vi "create_full_request_data.vi"(0 "llm_ollama_embedding in":refnum<class "llm_ollama_embedding.lvclass">, 5 "data":refnum<class "abstract_message_base.lvclass">[](array[class]), 11 "error in (no error)":errorcluster) -> (4 "llm_ollama_embedding out":refnum<class "llm_ollama_embedding.lvclass">, 6 "request_data":T1[](array[typedef]), 15 "error out":errorcluster)   [LabVIEW 2020, in "llm_ollama_embedding.lvclass"]
uses:
  llm_ollama_embedding.lvclass
  abstract_message_base/abstract_message_base.lvclass
  utils/request_Data.ctl
  llm_ollama_embedding.lvclass/llm_ollama_embedding.ctl
  message_text/message_text.lvclass
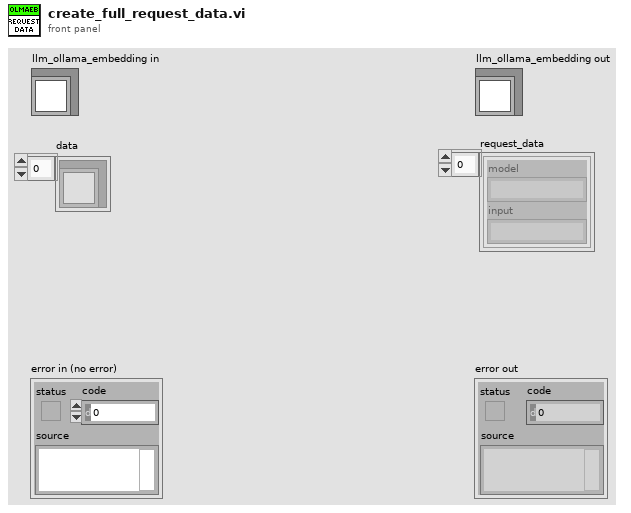
[diagram p1: front panel]
types:
  T1 = typedef "llm_ollama_embedding.lvclass/request_Data.ctl" = cluster{"model":string, "input":string}
  T2 = typedef "message_text.lvclass/message.ctl" = cluster{"role":string, "content":string[]}
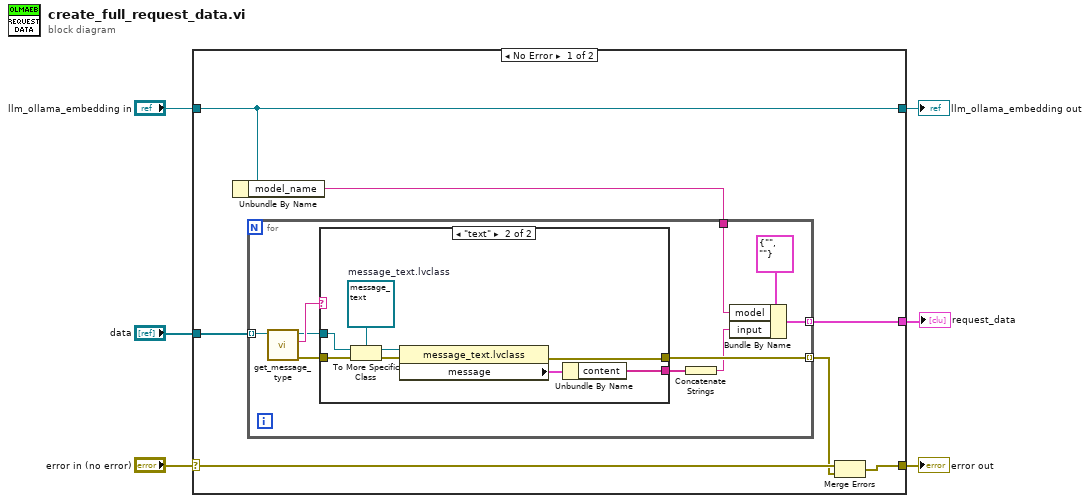
[diagram p0: block diagram]
diagram:
  n1 = case shown="No Error" "error in (no error)" {
    selector: "error in (no error)" -> [w13 w34]
    tunnel: [w10 w34] -> w5
    tunnel: [w11 w33] -> w3
    tunnel: "llm_ollama_embedding in" -> [w11 w33]
    tunnel: "data" -> [w12 _]
    tunnel: [w7 _] -> w1
    frame No Error {
      n2 = Unbundle By Name(w11) -> ("model_name"=w8:string)
      n3 = for {
        tunnel: w12 -> [w23] mode=indexing
        tunnel: [w19] -> w9 mode=indexing
        tunnel: w8 -> [w17]
        tunnel: [w14] -> w7 mode=indexing
        n4 = call-dynamic "get_message_type.vi"("abstract_message_base in"=w23) -> ("error out"=w20:errorcluster, "Type"=w22:string, "abstract_message_base out"=w21:refnum<class "abstract_message_base.lvclass">)  [unwired: 8 in]
        n5 = case shown="\"text\"" w22 {
          tunnel: w21 -> [_ w31]
          tunnel: w20 -> [w24 w32]
          tunnel: [w24 w27] -> w19
          tunnel: [_ w25] -> w18
          frame Default {
          }
          frame "text" {
            w30 = refnum<class "message_text.lvclass"> refnum  # message_text.lvclass
            n6 = To More Specific Class(target class=w30, reference=w31, error in=w32) -> (specific class reference=w29:refnum<class "message_text.lvclass">, error out=w28:errorcluster)
            n7 = property class="message_text.lvclass"(reference=w29, error in=w28) -> (error out=w27:errorcluster, "message"=w26:T2)  [unwired: 1 out]
            n8 = Unbundle By Name(w26) -> ("content"=w25:string[])
          }
        }
        n9 = Concatenate Strings(w18) -> (w16:string)
        n10 = Bundle By Name(cluster=T1 {"model"="", "input"=""} ("request data"), "model"=w17, "input"=w16) -> (w14:T1)
      }
      n11 = Merge Errors(w13, w9) -> (w10:errorcluster)
    }
    frame Error {
    }
  }
  "error out" <- w5
  "llm_ollama_embedding out" <- w3
  "request_data" <- w1
